vi "Initialaze.vi"(5 "Tree.lvclass":refnum<class "Tree.lvclass">, 10 "Use History (T)":bool=TRUE, 11 "Tree Refnum":refnum<vi>) -> (0 "Error":errorcluster, 3 "Tree out":refnum<class "Tree.lvclass">)   [LabVIEW 2021, in "Tree.lvlib" / "Tree.lvclass"]
uses:
  Tree.lvclass
  Tree.lvclass/Tree.ctl
  Private/TreeController.vi
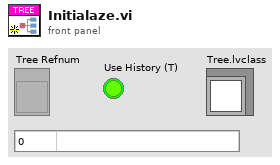
[diagram p1: front panel]
types:
  T1 = cluster{"0x01 Record modifications":bool, "0x02 Open templates for editing":bool, "0x04 Prompt user to save changes":bool, "0x08 Prepare for reentrant run":bool, "0x10 Prompt to find missing subVIs":bool, "0x20 Hide loading dialog box":bool, "0x40 Enable simultaneous calls on reentrant VIs":bool, "0x80 Prepare for call-and-forget":bool, "0x100 Prepare for call-and-collect":bool}
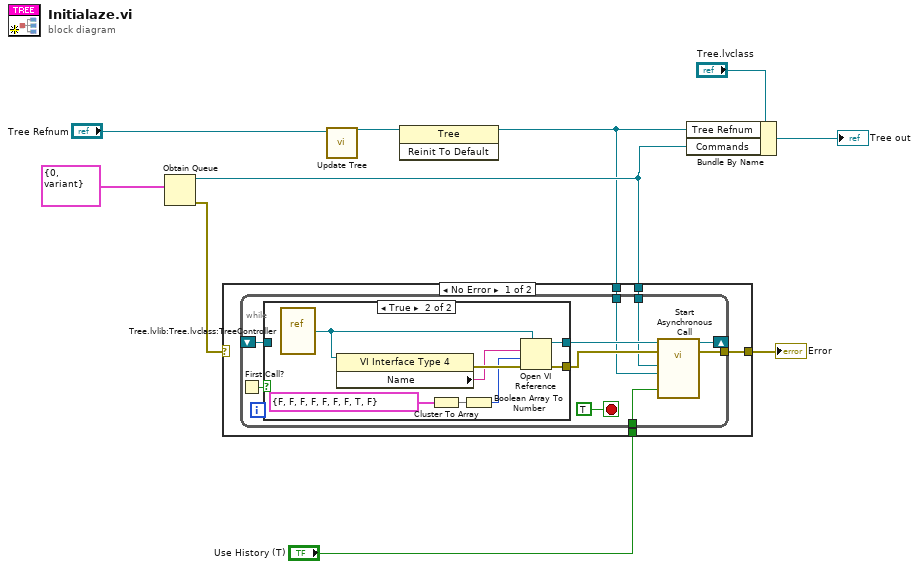
[diagram p0: block diagram]
diagram:
  n1 = Obtain Queue(element data type=cluster{"Tag":u8, "Value":variant} {"Tag"=0, "Value"=variant}) -> (queue out=w5:refnum<queue>, error out=w4:errorcluster)  [unwired: 4 in, 1 out]
  n2 = call "Update Tree.vi"("Tree Refnum"="Tree Refnum") -> ("Tree Refnum"=w1:refnum<vi>)  [unwired: 7 in, 3 out]
  n3 = invoke class="Tree" method="Reinit To Default"(reference=w1) -> (reference out=w3:refnum<vi>)  [unwired: 2 in, 2 out]
  n4 = case shown="No Error" w4 {
    selector: w4 -> [_ w34]
    tunnel: w5 -> [w14 _]
    tunnel: w3 -> [w13 _]
    tunnel: [w12 w34] -> w2
    tunnel: "Use History (T)" -> [w11 _]
    frame No Error {
      n5 = while {
        shift-right: [w19] -> _
        shift-left: _ -> [w21]
        tunnel: w14 -> [w18]
        tunnel: w13 -> [w17]
        tunnel: [w16] -> w12
        tunnel: w11 -> [w15]
        stop <- TRUE stop-if-true
        n6 = First Call?() -> (First Call?: T/F=w23:bool)
        n7 = case shown="True" w23 {
          tunnel: [_ w33] -> w24
          tunnel: [w25 w32] -> w22
          tunnel: w21 -> [w25 _]
          frame False {
          }
          frame True {
            n8 = vi-ref "Tree.lvlib:Tree.lvclass:TreeController.vi"() -> (w29:refnum<vi>)
            n9 = property class="VI Interface Type 4"(reference=w29) -> (error out=w31:errorcluster, "Name"=w30:string)  [unwired: 1 in, 1 out]
            n10 = Cluster To Array(cluster=T1 {"0x01 Record modifications"=FALSE, "0x02 Open templates for editing"=FALSE, "0x04 Prompt user to save changes"=FALSE, "0x08 Prepare for reentrant run"=FALSE, "0x10 Prompt to find missing subVIs"=FALSE, "0x20 Hide loading dialog box"=FALSE, "0x40 Enable simultaneous calls on reentrant VIs"=FALSE, "0x80 Prepare for call-and-forget"=TRUE, "0x100 Prepare for call-and-collect"=FALSE} ("options")) -> (array=w27:bool[])
            n11 = Boolean Array To Number(Boolean array=w27) -> (number=w26:i32)
            n12 = Open VI Reference(type specifier VI Refnum (for type only)=w29, vi path=w30, options=w26, error in (no error)=w31) -> (vi reference=w32:refnum<vi>, error out=w33:errorcluster)  [unwired: 2 in]
          }
        }
        n13 = call-by-ref "Start Asynchronous Call"(reference=w22, error in=w24, "SaveHistory"=w15, "Tree Refnum"=w17, "Commands"=w18) -> (reference out=w19:refnum<vi>, error out=w16:errorcluster)  [unwired: 9 in]
      }
    }
    frame Error {
    }
  }
  "Error" <- w2
  n14 = Bundle By Name(cluster="Tree.lvclass", "Tree Refnum"=w3, "Commands"=w5) -> (→"Tree out":refnum<class "Tree.lvclass">)
